vi "Save.vi"(8 "error in (no error)":errorcluster, 9 "new command":string, 10 "Msg in":T1, 11 "FakePressureController in":refnum<class "DaqPad_NI6009.lvclass">) -> (0 "error out":errorcluster, 1 "Path":path, 2 "Msg out":T1, 3 "FakePressureController out":refnum<class "DaqPad_NI6009.lvclass">, 4 "new command":string)   [LabVIEW 2011, in "DaqPad_NI6009.lvclass"]
uses:
  DaqPad_NI6009.lvclass
  DriverMsg.ctl
  DaqPad_NI6009.lvclass/DaqPad_NI6009.ctl
panel:
  out "data":waveform(dbl)[](array[waveform])
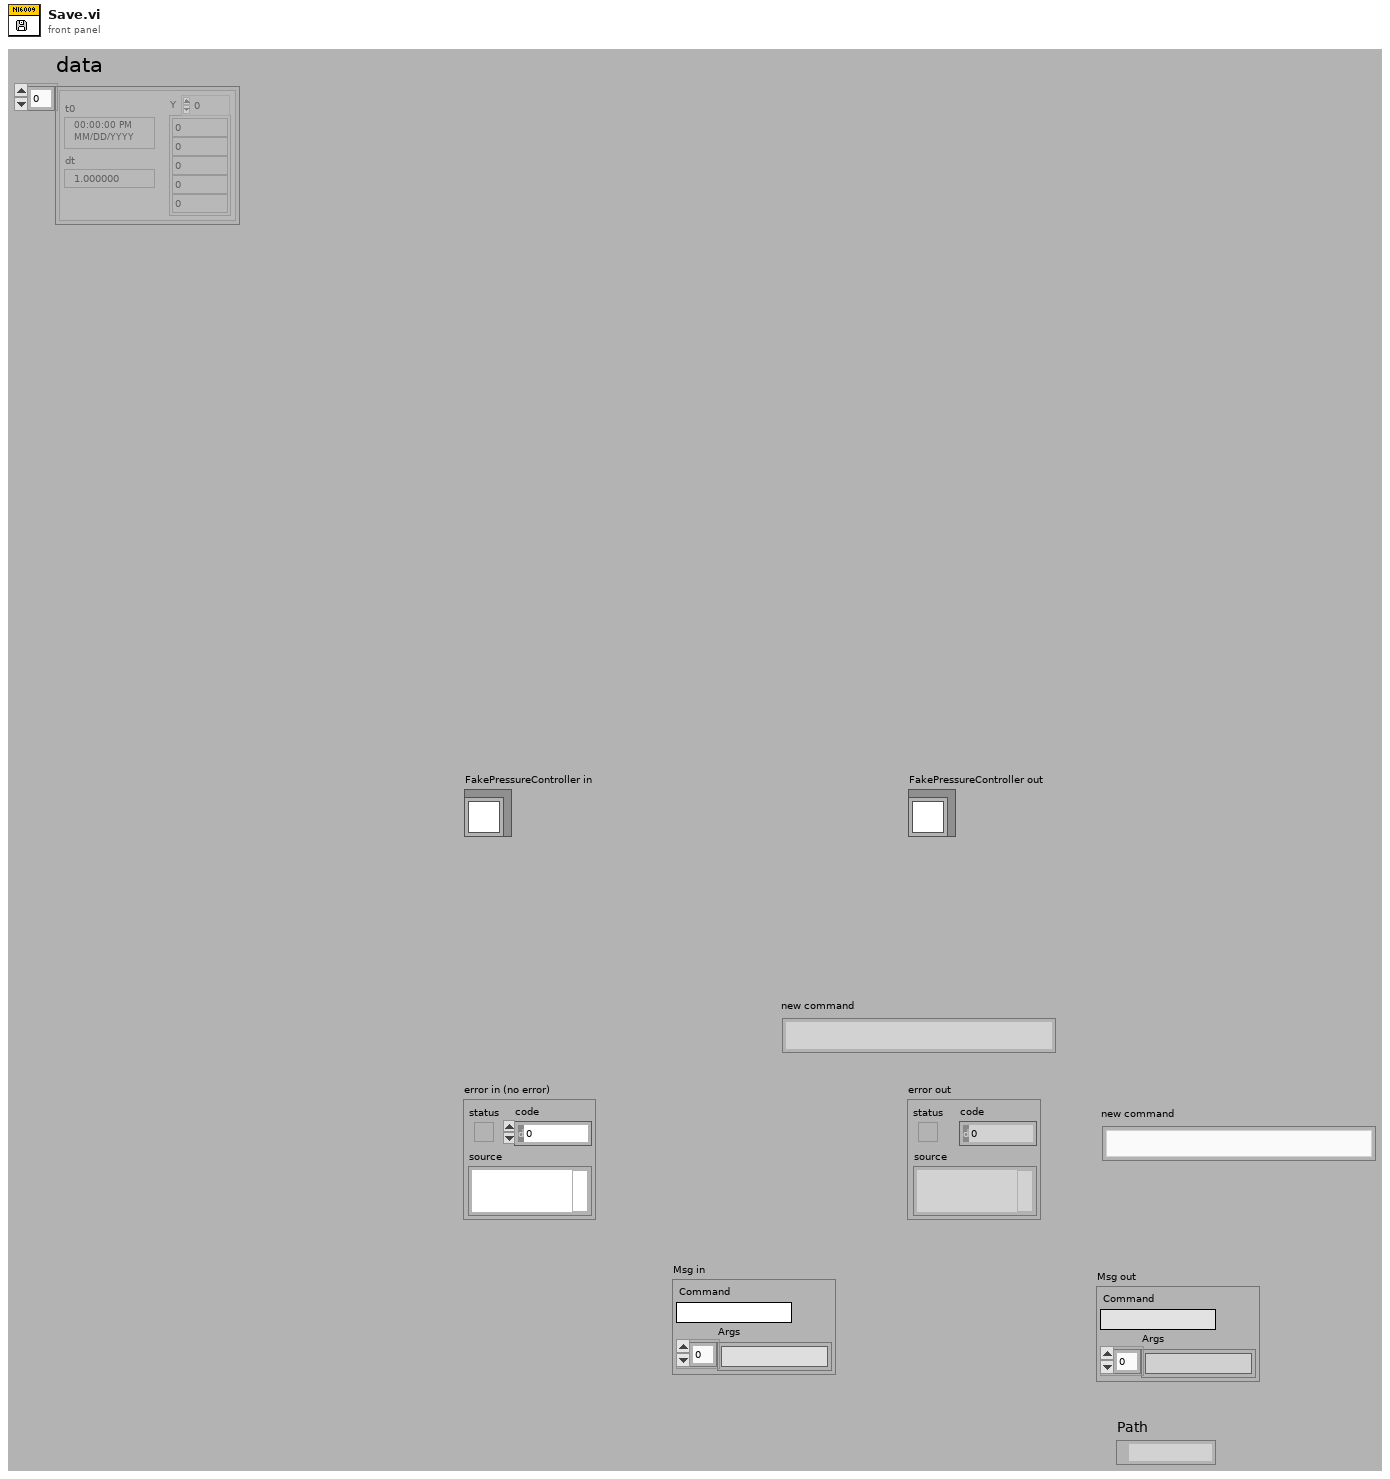
[diagram p1: front panel]
types:
  T1 = typedef "DriverMsg.ctl" = cluster{"Command":string, "Args":string[]}
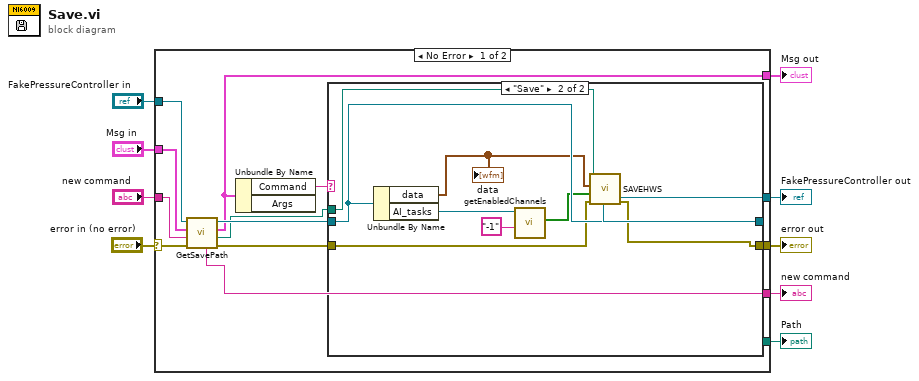
[diagram p0: block diagram]
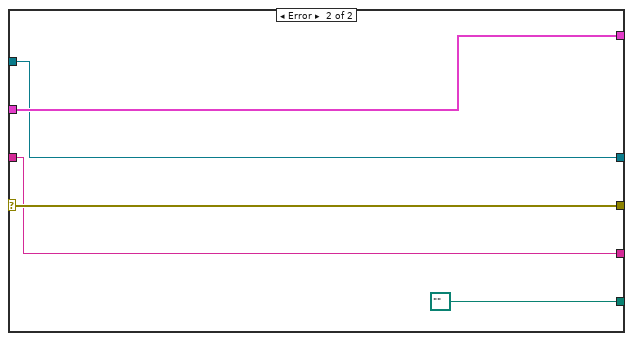
[diagram p3: hidden frame]
diagram:
  n1 = case shown="No Error" "error in (no error)" {
    selector: "error in (no error)" -> [w15 w36]
    tunnel: [w19 w36] -> w5
    tunnel: [_ path "" ("Path")] -> w1
    tunnel: [w13 w35] -> w6
    tunnel: [w20 w34] -> w8
    tunnel: "Msg in" -> [w17 w35]
    tunnel: "FakePressureController in" -> [w18 w34]
    tunnel: "new command" -> [w16 w32]
    tunnel: [w10 w32] -> w2
    frame No Error {
      n2 = call-dynamic "GetSavePath.vi"("error in (no error)"=w15, "new command"=w16, "Msg in"=w17, "BaseDriver in"=w18) -> ("error out"=w11:errorcluster, "Path"=w12:path, "Msg out"=w13:T1, "BaseDriver out"=w14:refnum<class "DaqPad_NI6009.lvclass">, "new command"=w10:string)  [unwired: 3 in]
      n3 = Unbundle By Name(w13) -> ("Command"=w21:string)  [unwired: 1 out]
      n4 = case shown="\"Save\"" w21 {
        tunnel: w14 -> [w23 w31]
        tunnel: [w23 w31] -> w20
        tunnel: w12 -> [_ w28]
        tunnel: w11 -> [w22 w26]
        tunnel: [w22 w25] -> w19
        frame Default {
        }
        frame "Save" {
          n5 = Unbundle By Name(w31) -> ("data"=w24:waveform(dbl)[], "AI_tasks"=w29:refnum<k21>)
          "data" <- w24
          n6 = call "getEnabledChannels.vi"("Channel (0.1.2.3)"="-1", "Refnum in"=w29) -> ("Enable (Array)"=w27:bool[])  [unwired: 6 in, 3 out]
          n7 = call "SAVEHWS.vi"("error in (no error)"=w26, "Enable (Array)"=w27, "data"=w24, "Destination HWS File"=w28) -> ("error out"=w25:errorcluster)  [unwired: 7 in]
        }
      }
    }
    frame Error {
    }
  }
  "error out" <- w5
  "FakePressureController out" <- w8
  "Path" <- w1
  "Msg out" <- w6
  "new command" <- w2
